vi "Open_Flywheel_PIDFs.vi"() -> (6 "output cluster":T1={"P Gain"=0.0, "I Gain"=0.0, "D Gain"=0.0, "F Gain"=0.0, "I Zone"=0.0, "Min Output"=0.0, "Max Output"=1.0})   [LabVIEW 2019]
uses:
  <vilib>/Utility/file.llb/Read Delimited Spreadsheet (string).vi
panel:
  in  "Cluster":T1
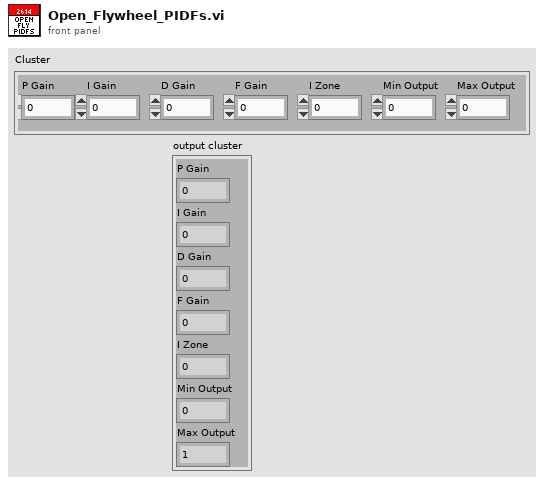
[diagram p1: front panel]
types:
  T1 = cluster{"P Gain":dbl, "I Gain":dbl, "D Gain":dbl, "F Gain":dbl, "I Zone":dbl, "Min Output":dbl, "Max Output":dbl}
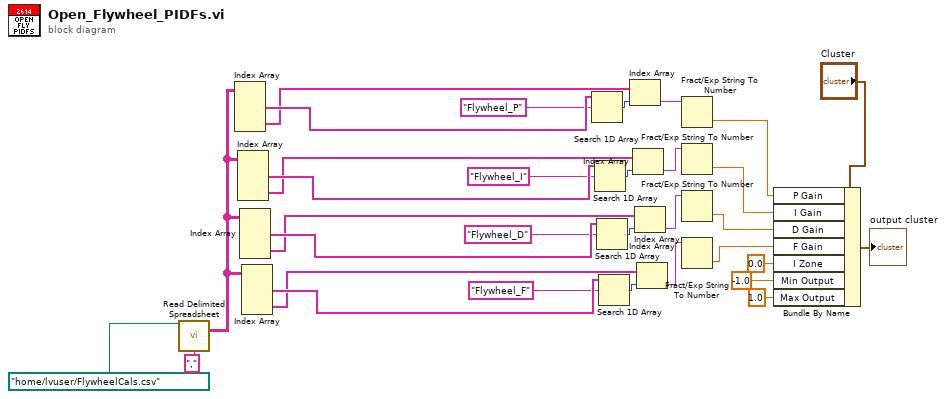
[diagram p0: block diagram]
diagram:
  n1 = call-poly <vilib>:"Read Delimited Spreadsheet.vi"("file path (dialog if empty)"=path "/home/lvuser/FlywheelCals.csv", "delimiter (\\t)"="," ("delimiter (\\t)")) -> ("all rows"=w10:string[][])  [unwired: 8 in, 5 out]
  n2 = Index Array(array=w10) -> (element #1=w30:string[], element #2=w29:string[])  [unwired: 4 in]
  n3 = Index Array(array=w10) -> (element #1=w25:string[], element #2=w24:string[])  [unwired: 4 in]
  n4 = Index Array(array=w10) -> (element #1=w20:string[], element #2=w19:string[])  [unwired: 4 in]
  n5 = Index Array(array=w10) -> (element #1=w15:string[], element #2=w14:string[])  [unwired: 4 in]
  n6 = Search 1D Array(1D array=w30, element="Flywheel_P") -> (index of element=w28:i32)  [unwired: 1 in]
  n7 = Search 1D Array(1D array=w25, element="Flywheel_I") -> (index of element=w23:i32)  [unwired: 1 in]
  n8 = Search 1D Array(1D array=w20, element="Flywheel_D") -> (index of element=w18:i32)  [unwired: 1 in]
  n9 = Search 1D Array(1D array=w15, element="Flywheel_F") -> (index of element=w13:i32)  [unwired: 1 in]
  n10 = Index Array(array=w29, index=w28) -> (element=w26:string)
  n11 = Index Array(array=w24, index=w23) -> (element=w21:string)
  n12 = Index Array(array=w19, index=w18) -> (element=w16:string)
  n13 = Index Array(array=w14, index=w13) -> (element=w11:string)
  n14 = Fract/Exp String To Number(string=w26) -> (number=w8:dbl)  [unwired: 3 in, 1 out]
  n15 = Fract/Exp String To Number(string=w21) -> (number=w7:dbl)  [unwired: 3 in, 1 out]
  n16 = Fract/Exp String To Number(string=w16) -> (number=w6:dbl)  [unwired: 3 in, 1 out]
  n17 = Fract/Exp String To Number(string=w11) -> (number=w5:dbl)  [unwired: 3 in, 1 out]
  n18 = Bundle By Name(cluster="Cluster", "P Gain"=w8, "I Gain"=w7, "D Gain"=w6, "F Gain"=w5, "I Zone"=0.0, "Min Output"=-1.0, "Max Output"=1.0) -> (→"output cluster":T1)
